vi "Read Steps from File.vi"(8 "error in (no error)":errorcluster, 11 "Macro in":refnum<class "Macro.lvclass">) -> (0 "error out":errorcluster, 3 "Macro out":refnum<class "Macro.lvclass">)   [LabVIEW 2020, in "MacroAssert.lvlib" / "Macro.lvclass"]
uses:
  Macro.lvclass
  Macro.lvclass/Macro.ctl
  Step/Step.lvclass
  <vilib>/Utility/config.llb/NI_LVConfig.lvlib
  MacroAssert.lvlib
  CTLs/Step Type V3.ctl
  <vilib>/Utility/config.llb/Read Key (String).vi
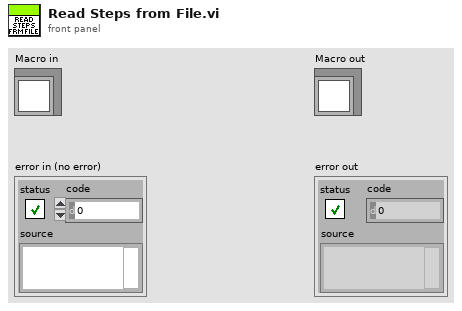
[diagram p1: front panel]
types:
  T1 = typedef "MacroAssert.lvlib/Step Type V3.ctl" = enum16{"Mouse Action", "Keyboard Action", "Window Action", "Timing Action", "Boolean Assertion", "Numeric Assertion", "String Assertion", "Image Assertion"}
  T2 = typedef "NI_LVConfig.lvlib/Config Data RefNum.ctl" = refnum<k1>
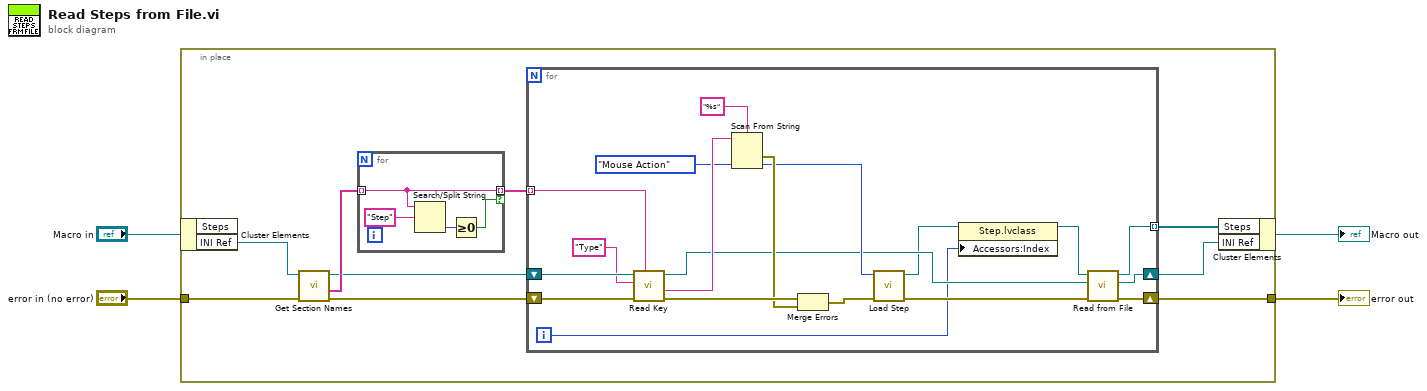
[diagram p0: block diagram]
diagram:
  n1 = in-place {
    in-place-border: "error in (no error)" -> [w12]
    in-place-border: [w7] -> w1
    n2 = in-place-cluster #1("Macro in") -> ("INI Ref"=w11:T2)  [unwired: 1 out]
    n3 = call <vilib>:"Get Section Names.vi"("error in (no error)"=w12, "refnum"=w11) -> ("error out"=w10:errorcluster, "section names"=w13:string[], "refnum out"=w9:T2)  [unwired: 7 in]
    n4 = for {
      tunnel: w13 -> [w33] mode=indexing
      tunnel: [w33] -> w8 mode=indexing if=w34
      n5 = Search/Split String(string=w33, search string/char (-)="Step") -> (offset of match=w35:i32)  [unwired: 1 in, 2 out]
      n6 = Greater Or Equal To 0?(x=w35) -> (x >= 0?=w34:bool)
    }
    n7 = for {
      tunnel: w8 -> [w29] mode=indexing
      shift-right: [w19] -> w7
      shift-left: w10 -> [w32]
      shift-right: [w18] -> w6
      shift-left: w9 -> [w30]
      tunnel: [w14] -> w5 mode=indexing
      i -> [w17]
      n8 = call-poly <vilib>:"Read Key.vi"("section"=w29, "error in (no error)"=w32, "key"="Type", "refnum"=w30) -> ("error out"=w31:errorcluster, "value"=w26:string, "refnum out"=w20:T2)  [unwired: 4 in, 1 out]
      n9 = Scan From String(format string="%s", input string=w26, default 1=Step_Type_V3."Mouse Action" ("Step Type")) -> (error out=w24:errorcluster, output 1=w22:T1)  [unwired: 2 in, 2 out]
      n10 = Merge Errors(w31, w24) -> (w25:errorcluster)
      n11 = call "Load Step.vi"("error in (no error)"=w25, "Step Type"=w22) -> ("error out"=w21:errorcluster, "Step"=w16:refnum<class "Step.lvclass">)  [unwired: 8 in]
      n12 = property class="Step.lvclass"(reference=w16, "Accessors:Index"=w17) -> (reference out=w15:refnum<class "Step.lvclass">)  [unwired: 1 in, 1 out]
      n13 = call-dynamic "Read from File.vi"("error in (no error)"=w21, "INI Ref"=w20, "Step in"=w15) -> ("error out"=w19:errorcluster, "INI Ref out"=w18:T2, "Step out"=w14:refnum<class "Step.lvclass">)  [unwired: 6 in]
    }
    n14 = in-place-cluster #1("Steps"=w5, "INI Ref"=w6) -> (→"Macro out":refnum<class "Macro.lvclass">)
  }
  "error out" <- w1
